vi "LoG_Convolution_Pure_Labview-3.vi"(4 "Keep Nega-\ntive Values?":bool, 5 "error IN":errorcluster, 6 "[IN] Sigma":dbl min=0.1, 7 "[IN] Processed Image":T1, 8 "[IN] Source Image":T1) -> (0 "error out":errorcluster, 3 "[OUT] Processed Image":T1)   [LabVIEW 2013]
doc: "Convolution of image with LoG spatial mask\nBorders are mirrored\nImplementation with built-in spatial convolution mask"
uses:
  <vilib>/vision/Image Controls.llb/IMAQ Image.ctl
  <vilib>/vision/Image Controls.llb/IMAQ Rounding Mode.ctl
  <vilib>/vision/NI_Vision_Development_Module.lvlib
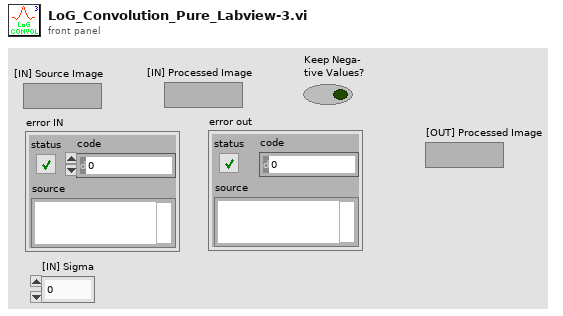
[diagram p1: front panel]
types:
  T1 = typedef "IMAQ Image.ctl" = refnum<image>
  T2 = typedef "IMAQ Rounding Mode.ctl" = enum16{"Optimize", "Truncate"}
  T3 = typedef "Image Type" = u32
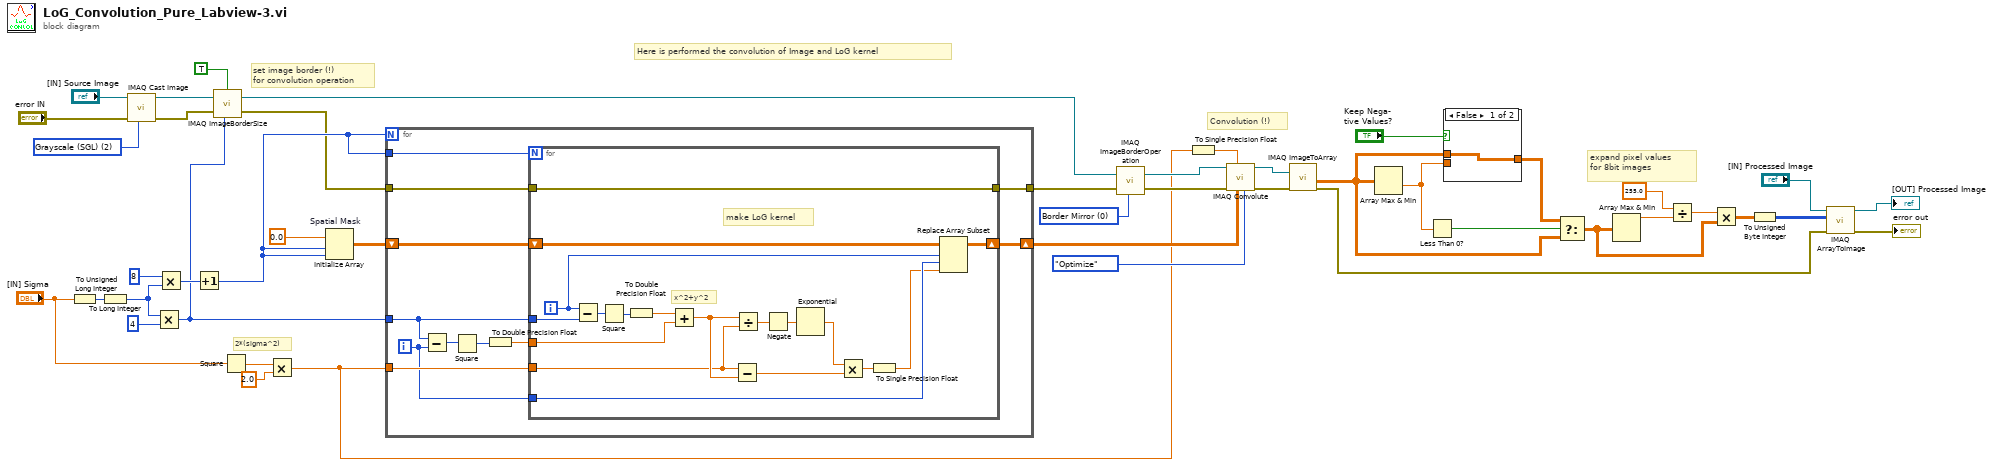
[diagram p0: block diagram]
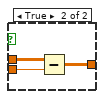
[diagram p2: hidden frame]
diagram:
  w26 = u32 0 items=["Border Mirror", "Border Copy", "Border Clear"] ("Function")
  w22 = T3 2 items=["Grayscale (U8)", "Grayscale (I16)", "Grayscale (SGL)", "Complex (CSG)", "RGB (U32)", "HSL (U32)", "RGB (U64)", "Grayscale (U16)"] ("Image Type")
  # "Convolution (!)"
  # "set image border (!) \nfor convolution operation"
  # "expand pixel values \nfor 8bit images"
  # "2*(sigma^2)"
  # "Here is performed the convolution of Image and LoG kernel"
  n1 = To Unsigned Long Integer(number="[IN] Sigma") -> (unsigned 32bit integer=w42:u32)
  n2 = To Long Integer(number=w42) -> (32bit integer=w41:i32)
  n3 = call "IMAQ Cast Image"("Image Type"=w22, "error in (no error)"="error IN", "Image Src"="[IN] Source Image") -> ("error out"=w17:errorcluster, "Image Dst Out"=w19:T1)  [unwired: 7 in]
  n4 = Multiply(x=w41, y=4) -> (x*y=w13:i32)
  n5 = Multiply(x=8, y=w41) -> (x*y=w20:i32)
  n6 = Increment(x=w20) -> (x+1=w16:i32)
  n7 = call "IMAQ ImageBorderSize"("Get/Set Status? (Set)"=TRUE, "Image"=w19, "Image border size in"=w13, "error in (no error)"=w17) -> ("Image Out"=w14:T1, "error out"=w15:errorcluster)  [unwired: 1 out]
  n8 = Square(x="[IN] Sigma") -> (x^2=w39:dbl)
  n9 = Multiply(x=w39, y=2.0) -> (x*y=w8:dbl)
  n10 = Initialize Array "Spatial Mask"(sgl 0.0 ("element"), w16, w16) -> (w43:sgl[][])
  n11 = for {
    N: w16 -> [_]
    shift-right: [w47] -> w12
    shift-left: w43 -> [w56]
    tunnel: w16 -> [w55]
    tunnel: w13 -> [w54]
    tunnel: w8 -> [w53]
    tunnel: w15 -> [w49]
    tunnel: [w46] -> w25
    i -> [w48]
    n12 = Subtract(x=w54, y=w48) -> (x-y=w52:i32)
    n13 = Square(x=w52) -> (x^2=w51:i32)
    n14 = To Double Precision Float(number=w51) -> (double precision float=w50:dbl)
    n15 = for {
      N: w55 -> [_]
      shift-right: [w60] -> w47
      shift-left: w56 -> [w63]
      tunnel: w54 -> [w74]
      tunnel: w53 -> [w68]
      tunnel: w50 -> [w70]
      tunnel: w49 -> [w59]
      tunnel: w48 -> [w61]
      tunnel: [w59] -> w46
      i -> [w62]
      # "make LoG kernel"
      # "x^2+y^2"
      n16 = Subtract(x=w62, y=w74) -> (x-y=w72:i32)
      n17 = Square(x=w72) -> (x^2=w73:i32)
      n18 = To Double Precision Float(number=w73) -> (double precision float=w71:dbl)
      n19 = Add(x=w71, y=w70) -> (x+y=w69:dbl)
      n20 = Subtract(x=w68, y=w69) -> (x-y=w65:dbl)
      n21 = Divide(x=w69, y=w68) -> (x/y=w67:dbl)
      n22 = Negate(x=w67) -> (-x=w66:dbl)
      n23 = Exponential(1:w66) -> (0:w64:dbl)
      n24 = Multiply(x=w64, y=w65) -> (x*y=w58:dbl)
      n25 = To Single Precision Float(number=w58) -> (single precision float=w57:sgl)
      n26 = Replace Array Subset(array=w63, new element=w57, index (row)=w62, index (col)=w61) -> (w60:sgl[][])
    }
  }
  n27 = call "IMAQ ImageBorderOperation"("Image"=w14, "Function"=w26, "error in (no error)"=w25) -> ("Image Out"=w23:T1, "error out"=w24:errorcluster)  [unwired: 2 in]
  n28 = To Single Precision Float(number=w8) -> (single precision float=w7:sgl)
  n29 = call "IMAQ Convolute"("Rounding Mode"=IMAQ_Rounding_Mode."Optimize", "Kernel"=w12, "Divider (kernel sum)"=w7, "error in (no error)"=w24, "Image Src"=w23) -> ("error out"=w34:errorcluster, "Image Dst Out"=w33:T1)  [unwired: 5 in]
  n30 = call "IMAQ ImageToArray"("error in (no error)"=w34, "Image"=w33) -> ("Image Pixels (Float)"=w2:sgl[][], "error out"=w27:errorcluster)  [unwired: 2 in, 3 out]
  n31 = Array Max & Min(array=w2) -> (min value=w5:sgl)  [unwired: 3 out]
  n32 = Less Than 0?(x=w5) -> (x < 0?=w32:bool)
  n33 = case shown="False" "Keep Nega-\ntive Values?" {
    tunnel: [w75 w78] -> w6
    tunnel: w5 -> [_ w77]
    tunnel: w2 -> [w75 w76]
    frame False {
    }
    frame True {
      n34 = Subtract(x=w76, y=w77) -> (x-y=w78:sgl[][])
    }
  }
  n35 = Select(t=w6, s=w32, f=w2) -> (s? t:f=w31:sgl[][])
  n36 = Array Max & Min(array=w31) -> (max value=w10:sgl)  [unwired: 3 out]
  n37 = Divide(x=sgl 255.0, y=w10) -> (x/y=w9:sgl)
  n38 = Multiply(x=w9, y=w31) -> (x*y=w30:sgl[][])
  n39 = To Unsigned Byte Integer(number=w30) -> (unsigned 8bit integer=w28:u8[][])
  n40 = call "IMAQ ArrayToImage"("error in (no error)"=w27, "Image Pixels (U8)"=w28, "Image"="[IN] Processed Image") -> ("error out"=→"error out":errorcluster, "Image Out"=→"[OUT] Processed Image":T1)  [unwired: 7 in]
